vi "Pause.vi"(8 "error in (no error)":errorcluster, 11 "Huber Settings In":T1) -> (0 "error out":errorcluster, 3 "Huber Settings Out":T1)   [LabVIEW 2018, in "Huber Ministat 230 TCU.lvlib"]
uses:
  Huber Ministat 230 TCU.lvlib
  Huber Settings.ctl
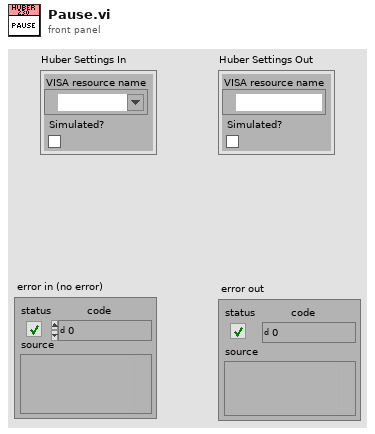
[diagram p1: front panel]
types:
  T1 = typedef "Huber Ministat 230 TCU.lvlib/Huber Settings.ctl" = cluster{"VISA resource name":refnum<visa-resource-name>, "Simulated?":bool}
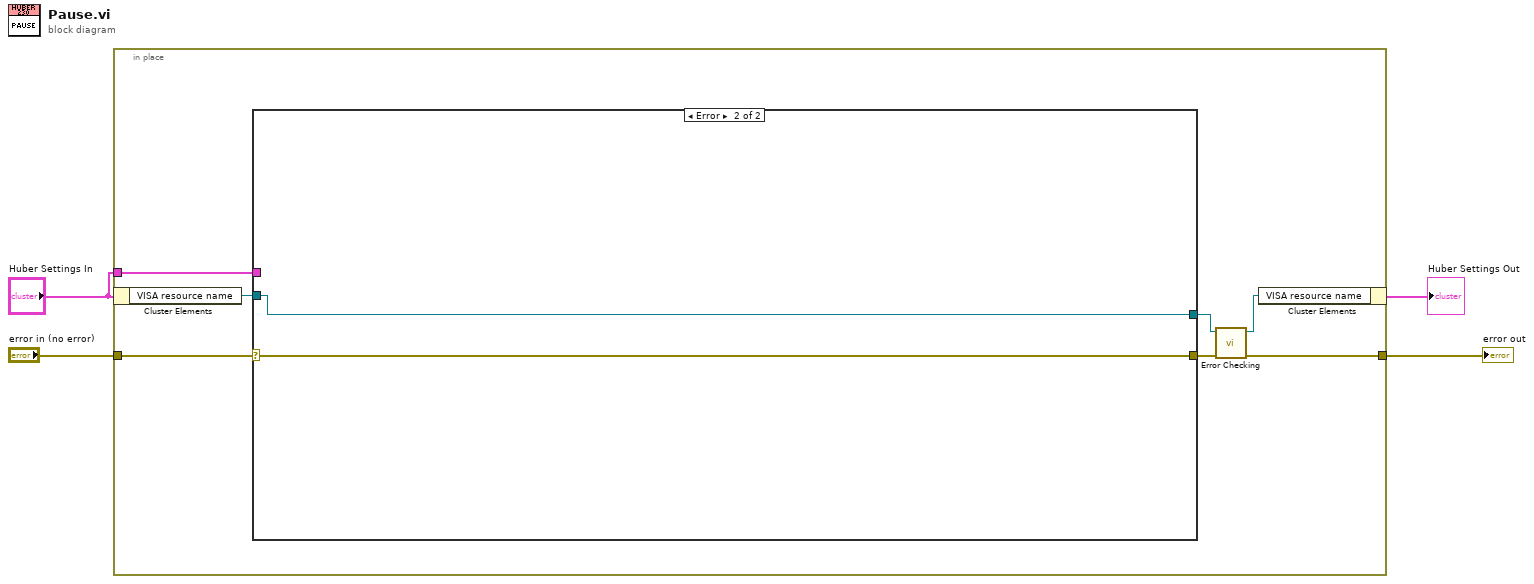
[diagram p0: block diagram]
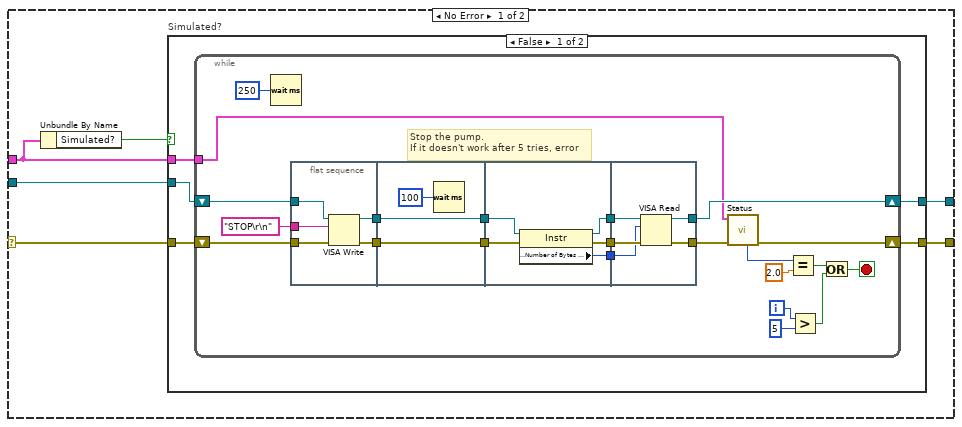
[diagram p2: hidden frame]
diagram:
  n1 = in-place {
    in-place-border: "error in (no error)" -> [w11]
    in-place-border: [w8] -> w3
    in-place-border: "Huber Settings In" -> [w7]
    n2 = in-place-cluster #1("Huber Settings In") -> ("VISA resource name"=w6:refnum<visa-resource-name>)
    n3 = case shown="Error" w11 {
      selector: w11 -> [w17 w66]
      tunnel: w7 -> [w13 _]
      tunnel: [w16 w66] -> w9
      tunnel: [w15 w65] -> w10
      tunnel: w6 -> [w12 w65]
      frame No Error {
        n4 = Unbundle By Name(w13) -> ("Simulated?"=w14:bool)
        n5 = case "Simulated?" shown="False" w14 {
          tunnel: w17 -> [w20 w64]
          tunnel: [w18 w64] -> w16
          tunnel: [w22 w63] -> w15
          tunnel: w12 -> [w21 w63]
          tunnel: w13 -> [w19 _]
          frame False {
            n6 = while {
              tunnel: w19 -> [w33]
              shift-right: [w36] -> w22
              shift-left: w21 -> [w35]
              shift-right: [w31] -> w18
              shift-left: w20 -> [w34]
              i -> [w26]
              stop <- w27 stop-if-true
              # "Stop the pump. \nIf it doesn't work after 5 tries, error"
              n7 = Wait (ms)(milliseconds to wait=u32 250) -> ()  [unwired: 1 out]
              n8 = flat-sequence {
                tunnel: "STOP\r\n" ("string") -> [w49]
                tunnel: [w48] -> w44
                tunnel: [w47] -> w43
                tunnel: w35 -> [w46]
                tunnel: w34 -> [w45]
                tunnel: w44 -> [w51]
                tunnel: w43 -> [w50]
                tunnel: [w51] -> w42
                tunnel: [w50] -> w41
                tunnel: [w55] -> w40
                tunnel: [w54] -> w39
                tunnel: [w53] -> w38
                tunnel: w42 -> [w57]
                tunnel: w41 -> [w56]
                tunnel: [w62] -> w32
                tunnel: [w61] -> w36
                tunnel: w40 -> [w60]
                tunnel: w39 -> [w59]
                tunnel: w38 -> [w58]
                frame #0 {
                  n9 = VISA Write(VISA resource name=w46, write buffer=w49, error in (no error)=w45) -> (VISA resource name out=w48:refnum<visa-resource-name>, error out=w47:errorcluster)  [unwired: 1 out]
                }
                frame #1 {
                  n10 = Wait (ms)(milliseconds to wait=u32 100) -> ()  [unwired: 1 out]
                }
                frame #2 {
                  n11 = property class="Instr"(reference=w57, error in=w56) -> (reference out=w55:refnum<visa-resource-name>, error out=w54:errorcluster, "Serial Settings:Number of Bytes at Serial Port"=w53:u32)
                }
                frame #3 {
                  n12 = VISA Read(VISA resource name=w60, byte count=w58, error in (no error)=w59) -> (VISA resource name out=w61:refnum<visa-resource-name>, error out=w62:errorcluster)  [unwired: 2 out]
                }
              }
              n13 = call "Status.vi"("error in (no error)"=w32, "Huber Settings"=w33) -> ("error out"=w31:errorcluster, "Temp"=w29:i32)  [unwired: 5 in, 3 out]
              n14 = Equal?(x=w29, y=2.0) -> (x = y?=w28:bool)
              n15 = Greater?(x=w26, y=5) -> (0:w24:bool)
              n16 = Or(x=w28, y=w24) -> (x .or. y?=w27:bool)
            }
          }
          frame True {
          }
        }
      }
      frame Error {
      }
    }
    n17 = call "Error Checking.vi"("error in (no error)"=w9, "VISA resource name"=w10) -> ("error out"=w8:errorcluster, "VISA resource name"=w5:refnum<visa-resource-name>)  [unwired: 7 in, 1 out]
    n18 = in-place-cluster #1("VISA resource name"=w5) -> (→"Huber Settings Out":T1)
  }
  "error out" <- w3
